vi "Get settings chain.vi"(8 "error in (no error)":errorcluster, 11 "BMCBase in":refnum<class "BMC.lvclass">) -> (0 "error out":errorcluster, 1 "class name":string[](array[string]), 2 "settings":variant[](array[variant]), 3 "BMCBase out":refnum<class "BMC.lvclass">)   [LabVIEW 2012, in "BMC.lvclass"]
doc: "Returns an array of variants containing the settings clusters of each class in the inheritance chain (lowest child class first), together with an array of all class names in the inheritance chain.\n\nFor classes without settings cluster, the settings chain contains empty variants."
uses:
  BMC.lvclass
  Murmex/LabVIEW/Murmex/Murmex/Murmex.lvclass
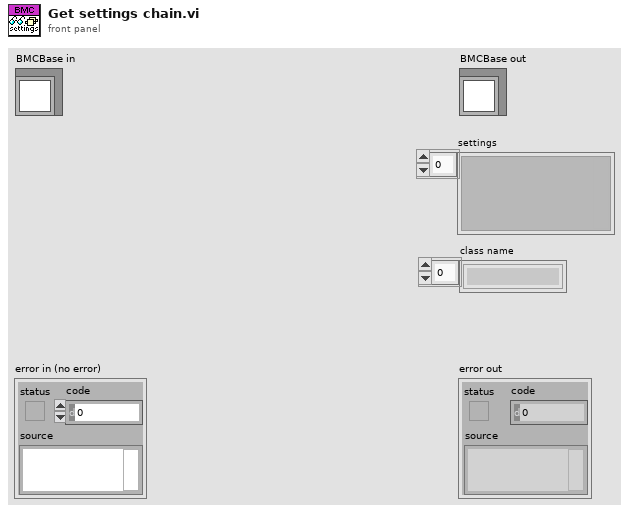
[diagram p1: front panel]
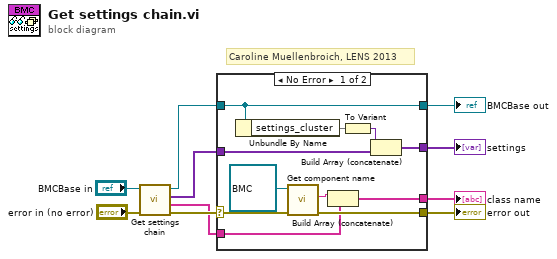
[diagram p0: block diagram]
diagram:
  # "Caroline Muellenbroich, LENS 2013"
  n1 = call-parent "Get settings chain.vi"("error in (no error)"="error in (no error)", "MurmexBase in"="BMCBase in") -> ("error out"=w8:errorcluster, "class name"=w6:string[], "settings"=w3:variant[], "MurmexBase out"=w4:refnum<class "BMC.lvclass">)  [unwired: 6 in]
  n2 = case shown="No Error" w8 {
    selector: w8 -> [w20 w24]
    tunnel: [w19 w24] -> w7
    tunnel: w6 -> [w17 w23]
    tunnel: [w16 w23] -> w5
    tunnel: w4 -> [w12 w25]
    tunnel: w3 -> [w13 w22]
    tunnel: [w12 w25] -> w2
    tunnel: [w11 w22] -> w1
    frame No Error {
      n3 = Unbundle By Name(w12) -> ("settings_cluster"=w15)
      n4 = call "Get component name.vi"("error in (no error)"=w20, "Murmex in"=refnum<class "BMC.lvclass"> refnum ("BMC")) -> ("error out"=w19:errorcluster, "component name"=w18:string)  [unwired: 7 in, 1 out]
      n5 = Build Array (concatenate)(w18, w17) -> (w16:string[])
      n6 = To Variant(anything=w15) -> (Variant=w14:variant)
      n7 = Build Array (concatenate)(w14, w13) -> (w11:variant[])
    }
    frame Error {
    }
  }
  "error out" <- w7
  "BMCBase out" <- w2
  "settings" <- w1
  "class name" <- w5
